vi "NI-845x_Config (SubVI).vi"(3 "error in (no error)":errorcluster, 4 "i2c configuration in":T2, 5 "Device in":T1) -> (0 "error out":errorcluster, 1 "i2c configuration out":T2, 2 "Device out":T1)   [LabVIEW 2017]
uses:
  <vilib>/ni845x/ni845x.llb/ni845xControl.ctl
  <vilib>/ni845x/ni845x.llb/ni845xI2cConfiguration.ctl
  <resource>/objmgr/NI845x.rc
panel:
  in  "Cancel":bool
  in  "Set":bool
  in  "I/O Voltage Level":i32(ring)=33 items=["3.3V"=33, "2.5V"=25, "1.8V"=18, "1.5V"=15, "1.2V"=12]
  in  "Use Internal I2C Pullup Resistor":bool
  in  "Clock Rate (kHz)":u16=100
  in  "Device":T1
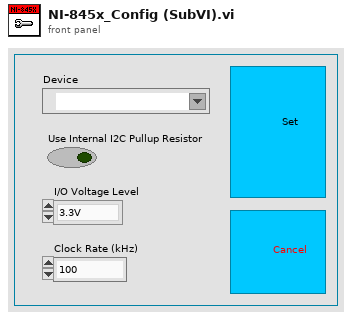
[diagram p1: front panel]
types:
  T1 = typedef "ni845xControl.ctl" = refnum<k21>
  T2 = typedef "ni845xI2cConfiguration.ctl" = refnum<k20>
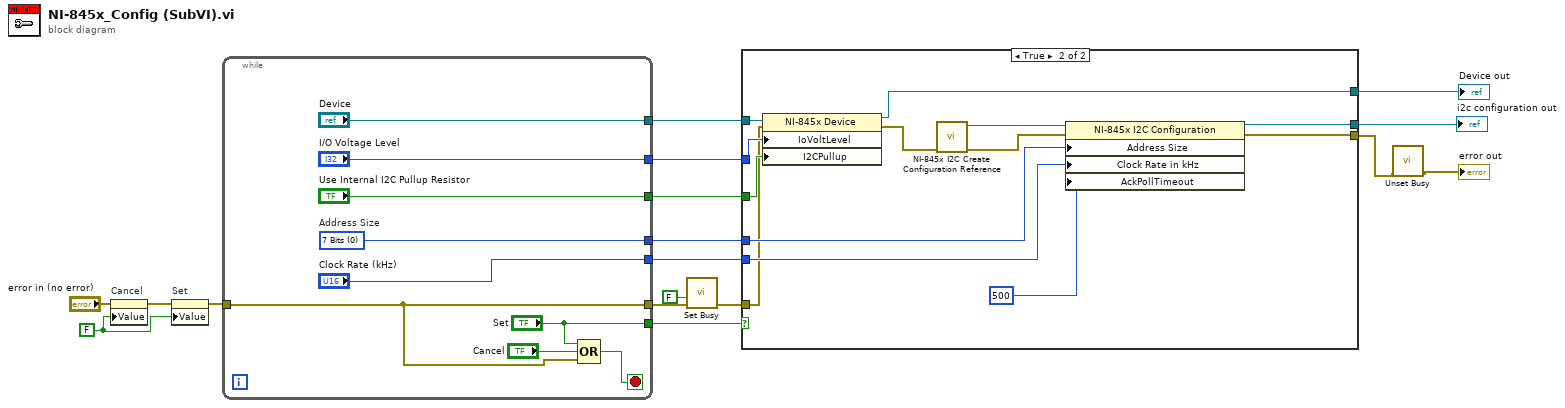
[diagram p0: block diagram]
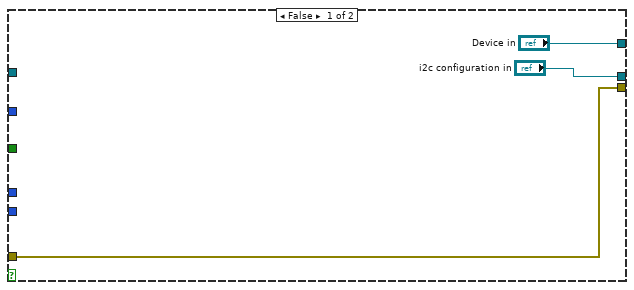
[diagram p2: hidden frame]
diagram:
  w3 = FALSE ("Cancel")
  n1 = property on="Cancel" class="Bool (strict)"(error in="error in (no error)", "Value"=w3) -> (error out=w4:errorcluster)  [unwired: 1 in, 1 out]
  n2 = property on="Set" class="Bool (strict)"(error in=w4, "Value"=w3) -> (error out=w1:errorcluster)  [unwired: 1 in, 1 out]
  n3 = while {
    tunnel: ["Clock Rate (kHz)"] -> w17
    tunnel: [w25] -> w16
    tunnel: ["Device"] -> w15
    tunnel: ["I/O Voltage Level"] -> w14
    tunnel: ["Use Internal I2C Pullup Resistor"] -> w13
    tunnel: ["Set"] -> w12
    tunnel: [w18] -> w8
    tunnel: w1 -> [w18]
    stop <- w21 stop-if-true
    w25 = 0 items=["7 Bits", "10 Bits"]  # Address Size
    n4 = Compound Arithmetic op=OR("Set", "Cancel", w18) -> (w21:bool)
  }
  n5 = call <vilib>:"Set Busy.vi"("error in (no error)"=w8, "disable click? (T)"=FALSE) -> ("error out"=w9:errorcluster)  [unwired: 8 in, 1 out]
  n6 = case shown="True" w12 {
    tunnel: w17 -> [_ w42]
    tunnel: w16 -> [_ w41]
    tunnel: w15 -> [_ w38]
    tunnel: w14 -> [_ w37]
    tunnel: w13 -> [_ w36]
    tunnel: w9 -> [w28 w34]
    tunnel: [w28 w33] -> w6
    tunnel: ["i2c configuration in" w32] -> w11
    tunnel: ["Device in" w31] -> w10
    frame False {
    }
    frame True {
      n7 = property on="Property Node" class="NI-845x Device"(reference=w38, error in=w34, "IoVoltLevel"=w37, "I2CPullup"=w36) -> (reference out=w31:T1, error out=w35:errorcluster)
      n8 = call <vilib>:"NI-845x I2C Create Configuration Reference.vi"("error in (no error)"=w35) -> ("error out"=w39:errorcluster, "i2c configuration"=w40:T2)  [unwired: 9 out]
      n9 = property class="NI-845x I2C Configuration"(reference=w40, error in=w39, "Address Size"=w41, "Clock Rate in kHz"=w42, "AckPollTimeout"=u16 500 ("ACK Poll Timeout")) -> (reference out=w32:T2, error out=w33:errorcluster)
    }
  }
  "i2c configuration out" <- w11
  "Device out" <- w10
  n10 = call <vilib>:"Unset Busy.vi"("error in (no error)"=w6) -> ("error out"=→"error out":errorcluster)  [unwired: 10 in]
